vi "Get Expected.vi"(11 "SDO Response Compare Strategy in":refnum<class "SDO Response Compare Strategy.lvclass">) -> (2 "Expected Response Message":refnum<class "CANopen Response Message.lvclass">, 3 "SDO Response Compare Strategy out":refnum<class "SDO Response Compare Strategy.lvclass">)   [LabVIEW 2024, in "CANopen Master.lvlib" / "SDO Response Compare Strategy.lvclass"]
uses:
  SDO Response Compare Strategy.lvclass
  CANopen Response/CANopen Response Message.lvclass
  SDO Response Compare Strategy.lvclass/SDO Response Compare Strategy.ctl
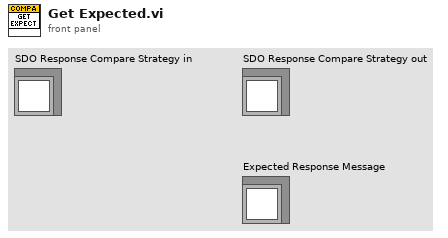
[diagram p1: front panel]
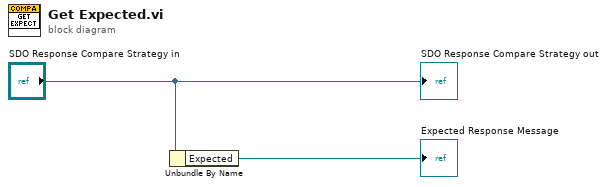
[diagram p0: block diagram]
diagram:
  n1 = Unbundle By Name("SDO Response Compare Strategy in") -> ("Expected"=→"Expected Response Message":refnum<class "CANopen Response Message.lvclass">)
  "SDO Response Compare Strategy out" <- "SDO Response Compare Strategy in"
